vi "Warmup.vi"(8 "System":string, 10 "Frequency Address":i16=8) -> ()   [LabVIEW 2024]
uses:
  <vilib>/Utility/file.llb/Write Delimited Spreadsheet (string).vi
panel:
  out "Warmup Graph":cluster{"Y":dbl[], "Y":dbl[]}[](graph)
  in  "Freq Counter Channel":enum16{"Channel 1", "Channel 2", "Channel 3"}(ring)
  out "StartTime(String)":string
  in  "DC_SN":string
  in  "Warmup X Data":string[](array[string])
  out "Cycle":i32
  in  "Warmup Y Data":string[](array[string])
  in  "Halt Run":bool=TRUE
  in  "Gatetime":u16(ring) items=["1", ".1", "10"]
  in  "Unit_Number":string
  in  "Work Order":string
  in  "Nominal Frequency":string
  in  "Enter":bool
  in  "Minutes":i32=1 min=1 max=180 step=1
  in  "Serial Number":string
  # "Please Enter Values \nFor Each Text Box"
  # "You must halt the run or let it finish before exiting"
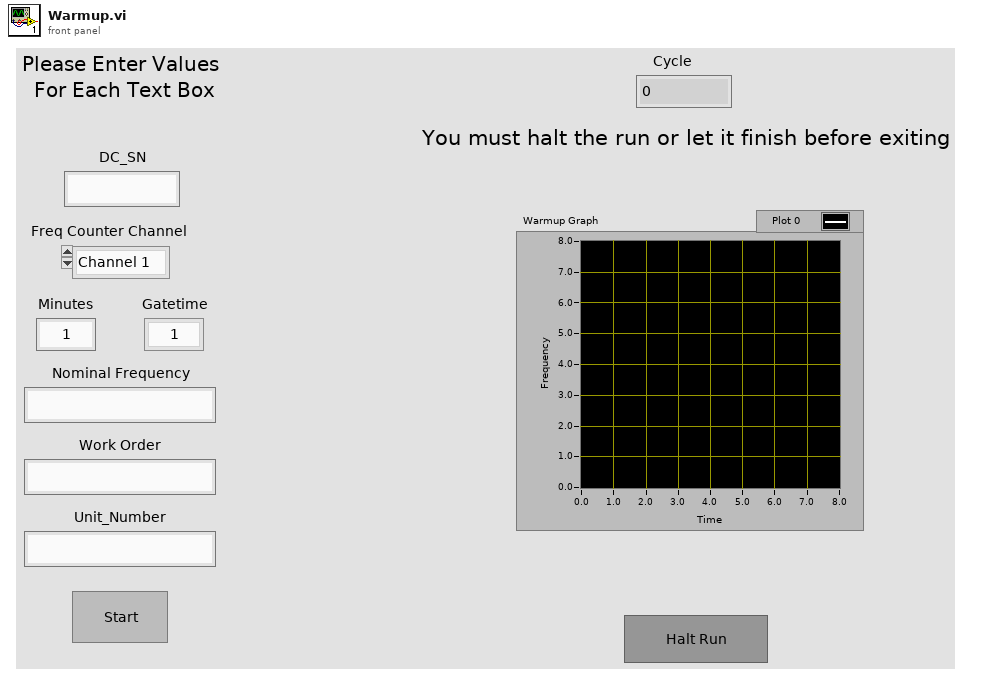
[diagram p1: front panel]
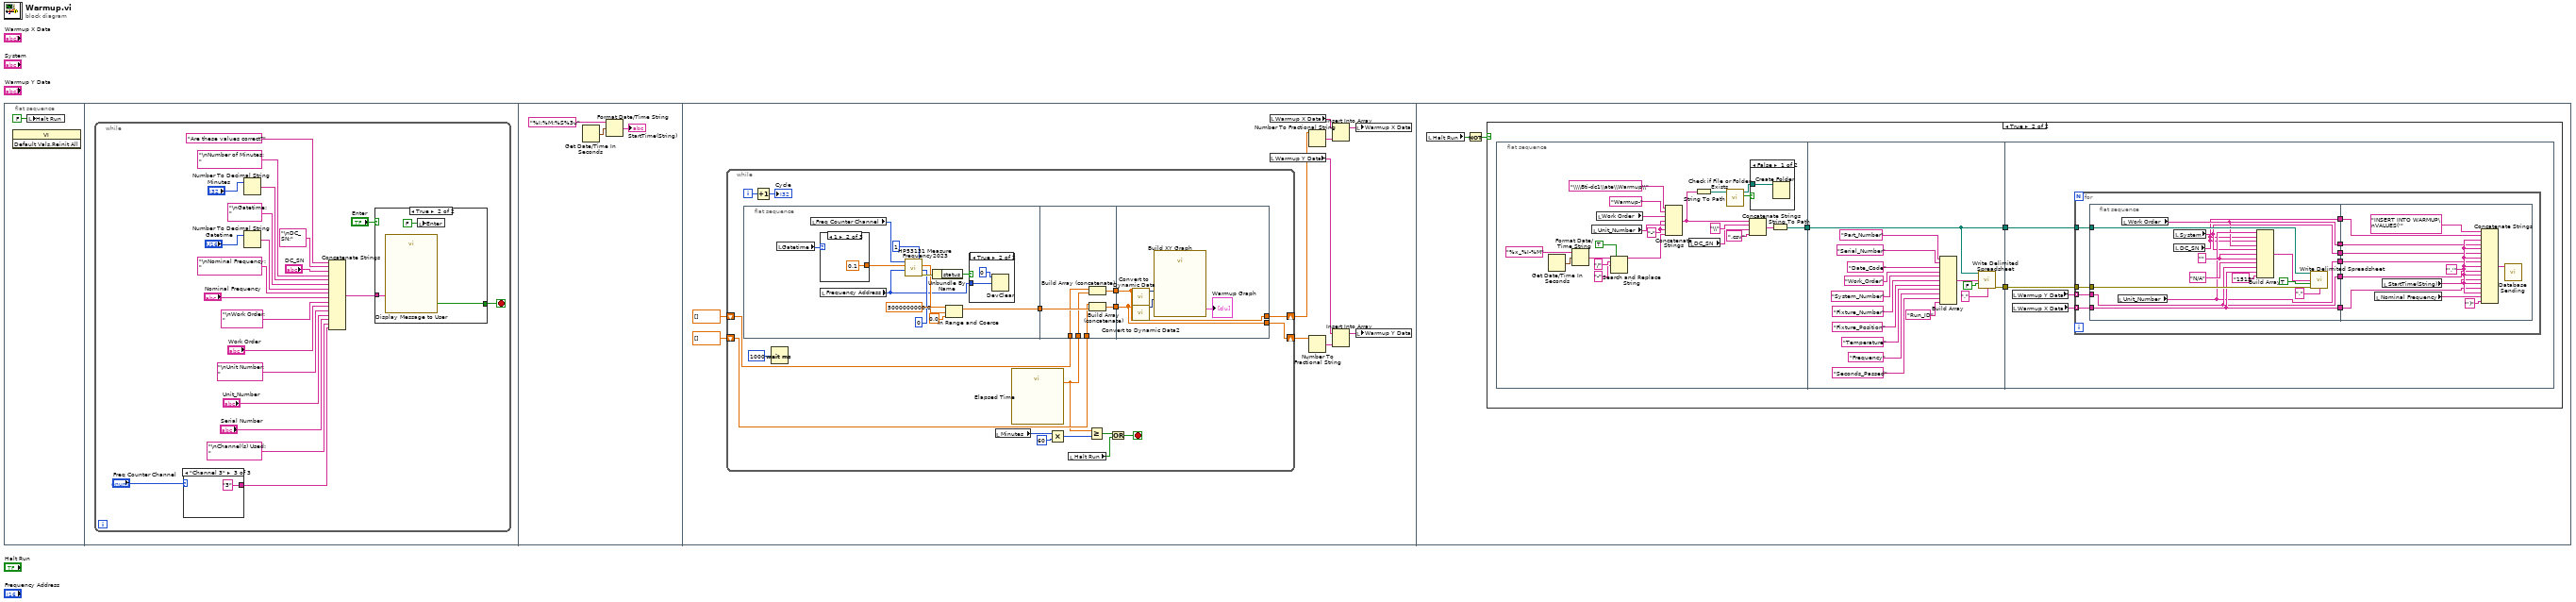
[diagram p0: block diagram]
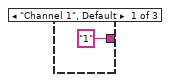
[diagram p2: hidden frame]
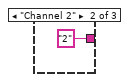
[diagram p3: hidden frame]
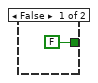
[diagram p4: hidden frame]
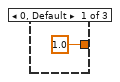
[diagram p5: hidden frame]
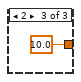
[diagram p6: hidden frame]
diagram:
  n1 = flat-sequence {
    frame #0 {
      n2 = invoke class="VI" method="Default Vals.Reinit All"() -> ()  [unwired: 3 in, 3 out]
      n3 = local write "Halt Run"(FALSE ("Halt Run")) -> ()
    }
    frame #1 {
      n4 = while {
        stop <- w22 stop-if-true
        n5 = case shown="\"Channel 3\"" "Freq Counter Channel" {
          tunnel: ["1" "2" "3"] -> w3
          frame "Channel 1", Default {
          }
          frame "Channel 2" {
          }
          frame "Channel 3" {
          }
        }
        n6 = Number To Decimal String(number="Minutes") -> (decimal integer string=w12:string)  [unwired: 1 in]
        n7 = Number To Decimal String(number="Gatetime") -> (decimal integer string=w10:string)  [unwired: 1 in]
        n8 = Concatenate Strings("Are these values correct?", "\nDC_SN:" ("string"), "DC_SN", "\nNumber of Minutes: " ("string"), w12, "\nGatetime: " ("string"), w10, "\nNominal Frequency: " ("string"), "Nominal Frequency", "\nWork Order: " ("string"), "Work Order", "\nUnit Number: " ("string"), "Unit_Number", "Serial Number", "\nChannel(s) Used: " ("string"), w3) -> (w20:string)
        n9 = case shown="True" "Enter" {
          tunnel: [FALSE w28] -> w22
          tunnel: w20 -> [_ w30]
          frame False {
          }
          frame True {
            n10 = call "Display Message to User"("Message"=w30) -> ("Yes"=w28:bool)  [unwired: 9 in, 1 out]
            n11 = local write "Enter"(FALSE ("Enter")) -> ()
          }
        }
      }
    }
    frame #2 {
      n12 = Get Date/Time In Seconds() -> (seconds since 1Jan1904=w31:timestamp)
      n13 = Format Date/Time String(time format string (%c)="%I:%M:%S%3u", seconds (now)=w31) -> (date/time string=→"StartTime(String)":string)  [unwired: 1 in]
    }
    frame #3 {
      n14 = while {
        shift-right: [w51] -> w35
        shift-left: dbl[] [] ("upper limit") -> [w59]
        shift-right: [w52] -> w36
        shift-left: dbl[] [] ("upper limit") -> [w58]
        i -> [w57]
        stop <- w44 stop-if-true
        n15 = flat-sequence {
          tunnel: [w72] -> w55
          tunnel: w59 -> [w82]
          tunnel: w58 -> [w81]
          tunnel: [w80] -> w54
          tunnel: w55 -> [w83]
          tunnel: [w79] -> w53
          tunnel: w47 -> [w78]
          tunnel: w54 -> [w85]
          tunnel: w53 -> [w84]
          tunnel: [w85] -> w52
          tunnel: [w84] -> w51
          frame #0 {
            n16 = local read "Gatetime"() -> (w63:u16)
            n17 = local read "Freq Counter Channel"() -> (w61:enum16{"Channel 1", "Channel 2", "Channel 3"})
            n18 = case shown="1" w63 {
              tunnel: [1.0 0.1 10.0] -> w62
              frame 0, Default {
              }
              frame 1 {
              }
              frame 2 {
              }
            }
            n19 = local read "Frequency Address"() -> (w64:i16)
            n20 = call "HP53131 Measure Frequency2023.vi"("GPIB Bus"=0, "Number of Readings"=1, "GPIB Address"=w64, "Gate Time"=w62, "Channel(1,2,3)"=w61) -> ("error out"=w71:errorcluster, "Frequency"=w65:dbl)  [unwired: 1 in]
            n21 = Unbundle By Name(w71) -> ("status"=w70:bool)
            n22 = In Range and Coerce(upper limit=5000000000.0, x=w65, lower limit=0.0) -> (coerced(x)=w72:dbl)  [unwired: 1 out]
            n23 = case shown="True" w70 {
              tunnel: w64 -> [_ w76]
              frame False {
              }
              frame True {
                n24 = DevClear(3:w76, 4:0 ("GPIB Bus")) -> ()  [unwired: 1 in, 2 out]
              }
            }
          }
          frame #1 {
            n25 = Build Array (concatenate)(w81, w78) -> (w80:dbl[])
            n26 = Build Array (concatenate)(w82, w83) -> (w79:dbl[])
          }
          frame #2 {
            n27 = call "Convert to Dynamic Data"("Array"=w85) -> ("Dynamic Data Type"=w87:dynamicdata)  [unwired: 3 in]
            n28 = call "Convert to Dynamic Data2"("Array"=w84) -> ("Dynamic Data Type"=w86:dynamicdata)  [unwired: 3 in]
            n29 = call "Build XY Graph"("Y Input"=w86, "X Input"=w87) -> ("XY Graph"=→"Warmup Graph":cluster{"X":dbl[], "Y":dbl[]}[])  [unwired: 8 in, 1 out]
          }
        }
        n30 = Increment(x=w57) -> (x+1=→"Cycle":i32)
        n31 = Wait (ms)(milliseconds to wait=u32 1000) -> ()  [unwired: 1 out]
        n32 = local read "Minutes"() -> (w50:i32)
        n33 = call "Elapsed Time"() -> ("Elapsed Time (s)"=w47:dbl)  [unwired: 12 in, 7 out]
        n34 = Multiply(x=w50, y=60) -> (x*y=w48:i32)
        n35 = local read "Halt Run"() -> (w45:bool)
        n36 = Greater Or Equal?(x=w47, y=w48) -> (x >= y?=w46:bool)
        n37 = Or(x=w46, y=w45) -> (x .or. y?=w44:bool)
      }
      n38 = local read "Warmup X Data"() -> (w39:string[])
      n39 = local read "Warmup Y Data"() -> (w40:string[])
      n40 = Number To Fractional String(number=w36) -> (F-format string=w37:string[])  [unwired: 3 in]
      n41 = Number To Fractional String(number=w35) -> (F-format string=w34:string[])  [unwired: 3 in]
      n42 = Insert Into Array(array=w39, new element=w37) -> (w38:string[])  [unwired: 1 in]
      n43 = Insert Into Array(array=w40, new element=w34) -> (w41:string[])  [unwired: 1 in]
      n44 = local write "Warmup X Data"(w38) -> ()
      n45 = local write "Warmup Y Data"(w41) -> ()
    }
    frame #4 {
      n46 = local read "Halt Run"() -> (w90:bool)
      n47 = Not(x=w90) -> (.not. x?=w89:bool)
      n48 = case shown="True" w89 {
        frame False {
        }
        frame True {
          n49 = flat-sequence {
            tunnel: [w94] -> w91
            tunnel: [w116] -> w93
            tunnel: [w117] -> w92
            tunnel: w91 -> [w116]
            tunnel: w93 -> [w135]
            tunnel: w92 -> [w134]
            frame #0 {
              w101 = "-" ("string")
              n50 = Get Date/Time In Seconds() -> (seconds since 1Jan1904=w112:timestamp)
              n51 = Format Date/Time String(time format string (%c)="%x_%I-%M" ("string"), seconds (now)=w112) -> (date/time string=w111:string)  [unwired: 1 in]
              n52 = local read "Unit_Number"() -> (w108:string)
              n53 = local read "Work Order"() -> (w109:string)
              n54 = Search and Replace String(replace all?=TRUE ("replace all? (F)"), input string=w111, search string="/", replace string="-" ("replace string (\"\")")) -> (result string=w110:string)  [unwired: 4 in, 3 out]
              n55 = Concatenate Strings("\\\\Bti-dc1\\ate\\Warmup\\" ("string"), "Warmup-" ("string"), w109, w101, w108, w101, w110) -> (w99:string)
              n56 = local read "DC_SN"() -> (w97:string)
              n57 = String To Path(string=w99) -> (path=w100:path)
              n58 = call <vilib>:"Check if File or Folder Exists.vi"("path"=w100) -> ("file or folder exists?"=w114:bool, "dup path"=w113:path)  [unwired: 8 in, 1 out]
              n59 = Concatenate Strings(w99, "\\" ("string"), w97, ".csv" ("string")) -> (w95:string)
              n60 = case shown="False" w114 {
                tunnel: w113 -> [w115 _]
                frame False {
                  n61 = Create Folder(path (use dialog)=w115) -> ()  [unwired: 2 in, 3 out]
                }
                frame True {
                }
              }
              n62 = String To Path(string=w95) -> (path=w94:path)
            }
            frame #1 {
              n63 = Build Array("Part_Number" ("string"), "Serial_Number" ("element"), "Date_Code" ("element"), "Work_Order" ("element"), "System_Number" ("element"), "Fixture_Number" ("element"), "Fixture_Position" ("element"), "Temperature" ("element"), "Frequency" ("element"), "Seconds_Passed" ("element"), "Run_ID" ("element")) -> (w131:string[])
              n64 = call-poly <vilib>:"Write Delimited Spreadsheet.vi"("file path (dialog if empty)"=w116, "1D data"=w131, "append to file? (new file:F)"=FALSE, "delimiter (\\t)"="," ("delimiter (\\t)")) -> ("error out"=w117:errorcluster)  [unwired: 10 in, 1 out]
            }
            frame #2 {
              n65 = local read "Warmup Y Data"() -> (w132:string[])
              n66 = local read "Warmup X Data"() -> (w133:string[])
              n67 = for {
                tunnel: w135 -> [w145]
                tunnel: w134 -> [w144]
                tunnel: w133 -> [w142] mode=indexing
                tunnel: w132 -> [w143] mode=indexing
                n68 = flat-sequence {
                  tunnel: w145 -> [w159]
                  tunnel: w144 -> [w153]
                  tunnel: w143 -> [w150]
                  tunnel: w142 -> [w151]
                  tunnel: [w151] -> w141
                  tunnel: [w150] -> w140
                  tunnel: [w149] -> w139
                  tunnel: [w148] -> w138
                  tunnel: [w147] -> w137
                  tunnel: [w146] -> w136
                  tunnel: w141 -> [w166]
                  tunnel: w140 -> [w165]
                  tunnel: w139 -> [w164]
                  tunnel: w138 -> [w163]
                  tunnel: w137 -> [w162]
                  tunnel: w136 -> [w161]
                  frame #0 {
                    w157 = "" ("element")
                    n69 = local read "Unit_Number"() -> (w149:string)
                    n70 = local read "Work Order"() -> (w147:string)
                    n71 = local read "System"() -> (w148:string)
                    n72 = local read "DC_SN"() -> (w146:string)
                    n73 = Build Array(w149, w146, w146, w147, w148, w157, w157, "N/A" ("element"), w150, w151, "1515" ("element")) -> (w154:string[])
                    n74 = call-poly <vilib>:"Write Delimited Spreadsheet.vi"("file path (dialog if empty)"=w159, "1D data"=w154, "append to file? (new file:F)"=TRUE, "error in (no error)"=w153, "delimiter (\\t)"="," ("delimiter (\\t)")) -> ()  [unwired: 9 in, 2 out]
                  }
                  frame #1 {
                    w170 = "','" ("element")
                    n75 = local read "Nominal Frequency"() -> (w167:string)
                    n76 = local read "StartTime(String)"() -> (w160:string)
                    n77 = Concatenate Strings("INSERT INTO WARMUP\nVALUES('" ("element"), w161, w170, w162, w170, w163, w170, w164, w170, w165, w170, w160, w170, w166, w170, w167, "')" ("Unit_Number")) -> (w168:string)
                    n78 = call "Database Sending.vi"("Command"=w168) -> ()  [unwired: 11 in]
                  }
                }
              }
            }
          }
        }
      }
    }
  }
